vi "Initialize and Register Sessions.vi"(8 "error in":errorcluster, 11 "sequence context":refnum<k7>) -> (0 "error out":errorcluster)   [LabVIEW 2021, in "NI-Switch Control Relay.lvlib"]
doc: "This VI will get called as part of the TestStand ProcessSetup sequence. It creates and registers all Switch sessions in the Session Mangement Service."
uses:
  NI-Switch Control Relay.lvlib
  <vilib>/gRPC/Generated APIs/ni/measurementlink/sessionmanagement/v1/RPC Messages/ni_measurementlink_PinMapContext.ctl
  <vilib>/Plug-In SDKs/Clients/Session Management V1/Session Reservation/Initialize and Close Session Behavior.ctl
  <vilib>/Plug-In SDKs/Clients/Session Management V1/Session Reservation/Session Reservation.lvclass
  <vilib>/Plug-In SDKs/TestStand/NI Pin Map TestStand.lvlib
  <vilib>/gRPC/Generated APIs/ni/measurementlink/sessionmanagement/v1/ni.measurementlink.sessionmanagement.v1.api.lvlib
  Source/Sessions/niSwitch/Session Management niSwitch.lvlib
  <instrlib>/niSwitch/niSwitch.llb/niSwitch Topologies.ctl
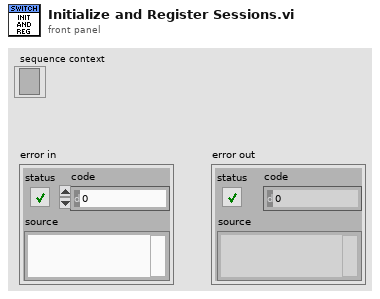
[diagram p1: front panel]
types:
  T1 = typedef "niSwitch Topologies.ctl" = string
  T2 = typedef "NI Session Management V1 Client.lvlib/Session Reservation.lvclass/Initialize and Close Session Behavior.ctl" = enum16{"Auto", "Initialize and Close", "Attach and Detach", "Initialize and Detach", "Attach and Close"}
  T3 = typedef "ni.measurementlink.sessionmanagement.v1.api.lvlib/ni_measurementlink_PinMapContext.ctl" = cluster{"pin_map_id":string, "sites":i32[]}
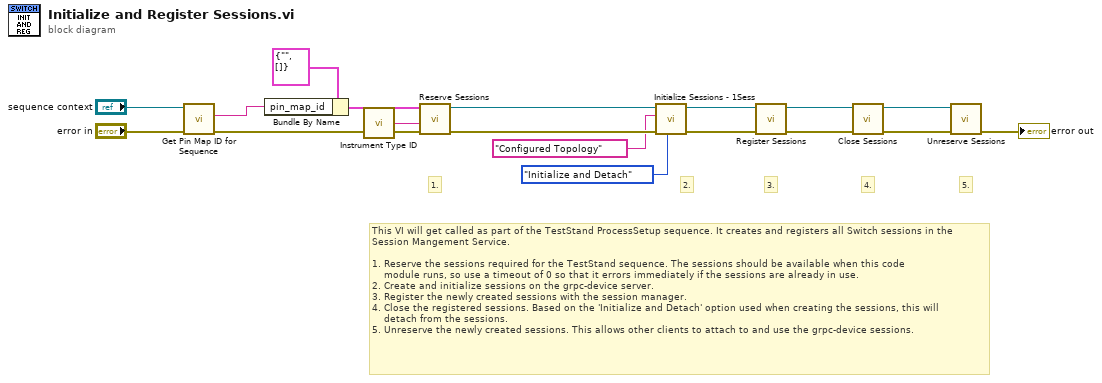
[diagram p0: block diagram]
diagram:
  # "4."
  # "5."
  # "3."
  # "2."
  # "1."
  # "This VI will get called as part of the TestStand ProcessSetup sequence. It creates and registers all Switch sessions in the\nSession Mangement Service.\n\n1. Reserve the sessions required for the TestStand sequence. The sessions should be available when this code\n    module runs, so use a timeout of 0 so that it errors immediately if the sessions are already in use.  \n2. Create and initialize sessions on the grpc-device server.\n3. Register the newly created sessions with the session manager.\n4. Close the registered sessions. Based on the 'Initialize and Detach' option used when creating the sessions, this will\n    detach from the sessions.\n5. Unreserve the newly created sessions. This allows other clients to attach to and use the grpc-device sessions."
  n1 = call <vilib>:"Get Pin Map ID for Sequence.vi"("error in"="error in", "sequence context in"="sequence context") -> ("error out"=w5:errorcluster, "pin map id"=w18:string)  [unwired: 7 in, 1 out]
  n2 = Bundle By Name(cluster=T3 {"pin_map_id"="", "sites"=[]} ("pin map context"), "pin_map_id"=w18) -> (w4:T3)
  n3 = call "Instrument Type ID.vi"() -> ("instrument type id"=w3:string)  [unwired: 5 in]
  n4 = call <vilib>:"Reserve Sessions.vi"("error in"=w5, "instrument type id"=w3, "pin map context"=w4) -> ("error out"=w14:errorcluster, "session reservation out"=w15:refnum<class "Session Reservation.lvclass">)  [unwired: 7 in]
  n5 = call "Initialize Sessions - 1Sess.vi"("initialize and close session behavior"=Initialize_and_Close_Session_Behavior."Initialize and Detach", "error in"=w14, "topology name"=T1 "Configured Topology", "session reservation in"=w15) -> ("error out"=w10:errorcluster, "session reservation out"=w13:refnum<class "Session Reservation.lvclass">)  [unwired: 4 in, 2 out]
  n6 = call <vilib>:"Register Sessions.vi"("error in"=w10, "session reservation in"=w13) -> ("error out"=w9:errorcluster, "session reservation out"=w12:refnum<class "Session Reservation.lvclass">)  [unwired: 8 in]
  n7 = call <vilib>:"Close Sessions.vi"("error in"=w9, "session reservation in"=w12) -> ("error out"=w8:errorcluster, "session reservation out"=w11:refnum<class "Session Reservation.lvclass">)  [unwired: 8 in]
  n8 = call <vilib>:"Unreserve Sessions.vi"("error in"=w8, "session reservation in"=w11) -> ("error out"=→"error out":errorcluster)  [unwired: 9 in]
